vi "Generate Random Color.vi"() -> (1 "Color":u32(colorbox))   [LabVIEW 2019]
doc: "This VI returns a random RGB color."
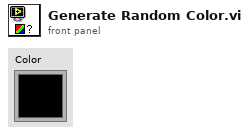
[diagram p1: front panel]
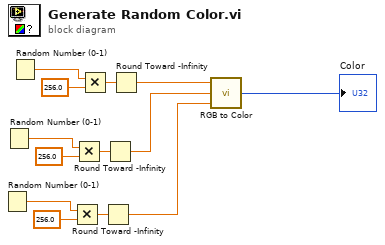
[diagram p0: block diagram]
diagram:
  n1 = Random Number (0-1)() -> (number: 0 to 1=w6:dbl)
  n2 = Random Number (0-1)() -> (number: 0 to 1=w7:dbl)
  n3 = Random Number (0-1)() -> (number: 0 to 1=w13:dbl)
  n4 = Multiply(x=w6, y=256.0) -> (x*y=w4:dbl)
  n5 = Multiply(x=w7, y=256.0) -> (x*y=w9:dbl)
  n6 = Multiply(x=w13, y=256.0) -> (x*y=w11:dbl)
  n7 = Round Toward -Infinity(1:w4) -> (0:w2:dbl)
  n8 = Round Toward -Infinity(1:w9) -> (0:w3:dbl)
  n9 = Round Toward -Infinity(1:w11) -> (0:w10:dbl)
  n10 = call <vilib>:"RGB to Color.vi"("B"=w2, "G"=w3, "R"=w10) -> ("Color"=→"Color":u32)
